vi "t.vi"() -> ()   [LabVIEW 2020]
uses:
  <vilib>/Platform/TimedLoop/XDataNode/timing_clust.ctl
  <vilib>/Platform/TimedLoop/XDataNode/nitl_modes.ctl
  <vilib>/Platform/TimedLoop/XDataNode/wakeup.ctl
  <vilib>/imath/engines/lvmath2/RunTimeEngine/ArithmeticOperatorToken/NIMS_ArithmeticOperator_plus.vi
  <instcachedir>/0/NIMS_ArithmeticOperator_plus_54468E2FAC2848C4BF0D457641184E60.lvgen/NIMS_ArithmeticOperator_plus_54468E2FAC2848C4BF0D457641184E60_012.vi
  <vilib>/imathl/engines/lvmath/Functions/Error Handling/Create Error.vi
  <instcachedir>/0/NIMS_NodeEndStatement_Output_53EC0D466D134D7ABD903AC30B43404B.lvgen/NIMS_NodeEndStatement_Output_53EC0D466D134D7ABD903AC30B43404B_005.vi
  <vilib>/imath/engines/lvmath2/RunTimeEngine/ErrorHandling/NIMS_Finalize Error.vi
  <vilib>/imath/engines/lvmath2/RunTimeEngine/Managers/WorkSpace/UID Generator.vi
  <vilib>/imath/engines/lvmath2/RunTimeEngine/RunTimeType/NIMS_RunTimeType_From StrictType (excl LVString).vi
  <instcachedir>/0/NIMS_RunTimeType_From StrictType (excl LVString)_283B1B2000484AAA8744D21CE97EA49F.lvgen/NIMS_RunTimeType_From StrictType (excl LVString)_283B1B2000484AAA8744D21CE97EA49F_000.vi
  <vilib>/imath/engines/lvmath2/RunTimeEngine/LocalVariableDefStatement/MC_LocalVariableDefStatement_Display.vi
  <vilib>/imath/engines/lvmath2/RunTimeEngine/Managers/SymbolTable/Clear UID.vi
  <instcachedir>/0/NIMS_NodeEndStatement_Output_53EC0D466D134D7ABD903AC30B43404B.lvgen/NIMS_NodeEndStatement_Output_53EC0D466D134D7ABD903AC30B43404B_001.vi
  <instcachedir>/0/NIMS_NodeEndStatement_Output_53EC0D466D134D7ABD903AC30B43404B.lvgen/NIMS_NodeEndStatement_Output_53EC0D466D134D7ABD903AC30B43404B_002.vi
  <vilib>/Platform/TimedLoop/XDataNode/XDataNode.xnode
  <vilib>/Platform/TimedLoop/XDataNode/XDNodeRunTimeDep.lvlib
  <vilib>/imath/engines/lvmath2/RunTimeEngine/Managers/SymbolTable/NIMS_WorkSpace.lvlib
panel:
  in  "保存路径":path=path "C:/Qmz/data1.bin"
  out "Swing":dbl[](graph)
  out "d_next":dbl
  out "y":dbl[][](array[numeric])
  out "添加的数组":dbl[][](array[numeric])
  out "x_next":dbl[](array[numeric])
  out "列数":i32
  out "行数":i32
  out "数组":dbl[](array[numeric])
  in  "PID/ARC":bool
  out "字符串":string="这是开环"
  in  "开环":bool=TRUE
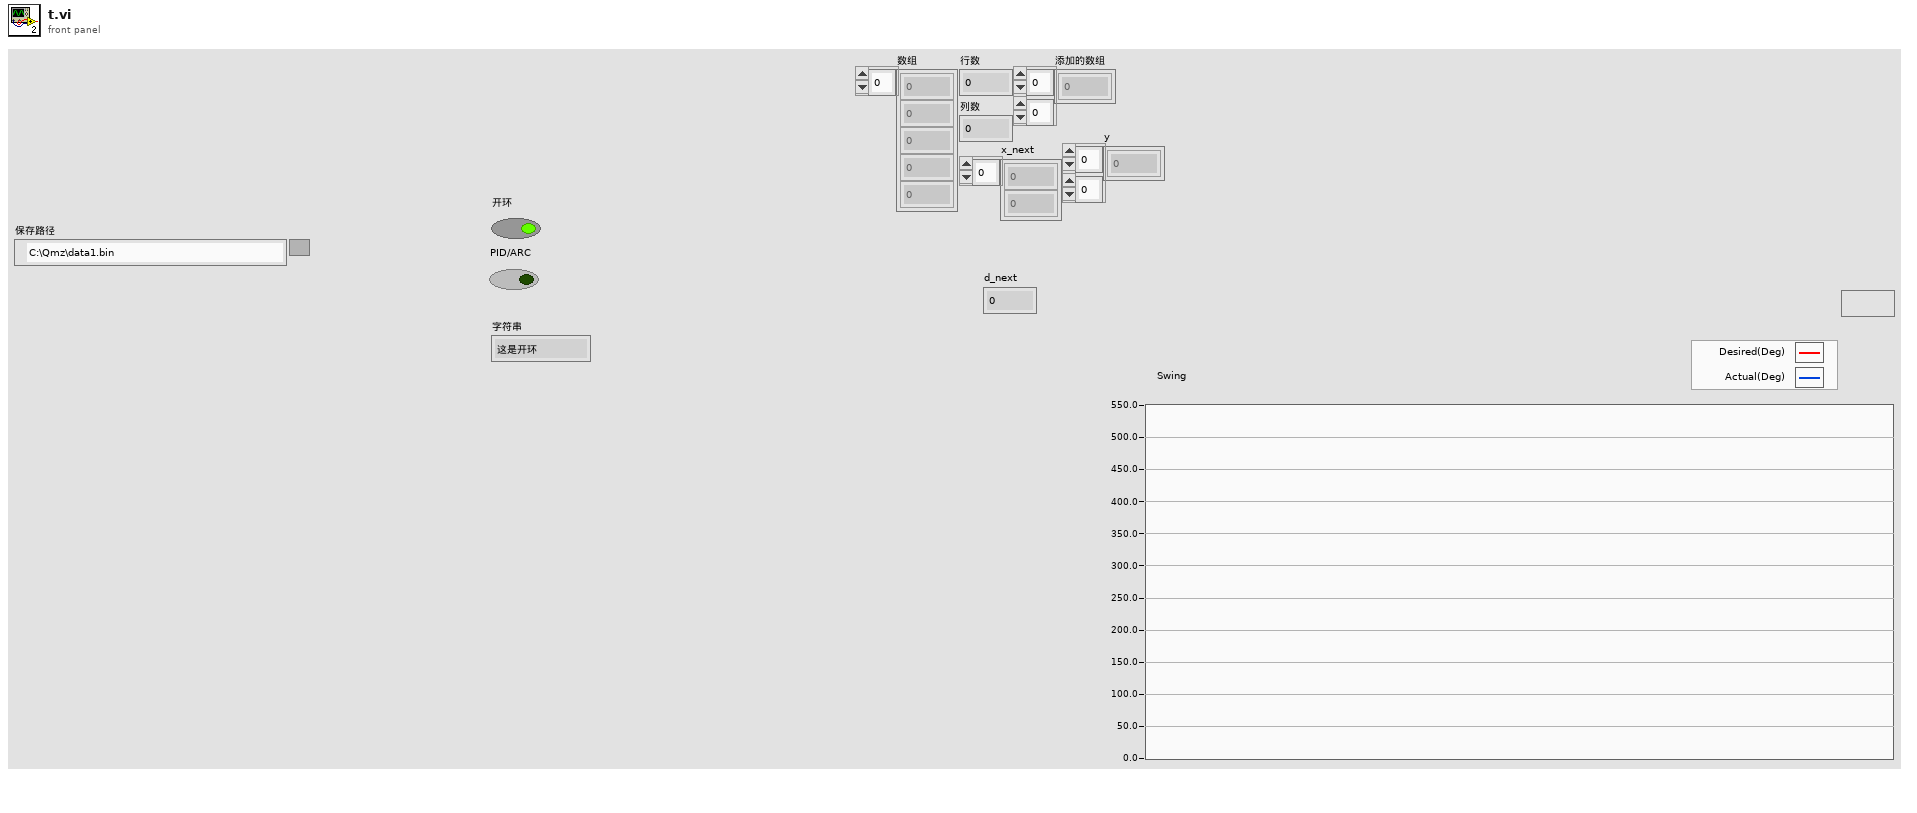
[diagram p1: front panel]
types:
  T1 = enum16{"open", "replace", "create", "open or create", "replace or create", "replace or create with confirmation"}
  T2 = typedef "XDNodeRunTimeDep.lvlib/timing_clust.ctl" = cluster{"Expected End [f-1]":u64, "Actual End [f-1]":u64, "Finished Late? [f-1]":bool, "Expected End [i-1]":u64, "Actual End [i-1]":u64, "Finished Late? [i-1]":bool, "Expected Start [i]":u64, "Actual Start [i]":u64, "Expected Start [f]":u64, "Actual Start [f]":u64, "Source Name":string, "Structure Name":string, "Period":i64, "Deadline":i64, "Offset":i64, "Start":i64, "Priority":i32, "Timeout":i32, "Mode":T3, "Wakeup Reason":T4, "Error":errorcluster, "Source Type":string, "Secondary Source Type":string, "Global End Time":u64, "Global Start Time":u64, "Frame Duration":u64, "Iteration Duration":u64, "Assigned CPU":i32, "I/O Scan Engine Mode":u32}
  T3 = typedef "XDNodeRunTimeDep.lvlib/nitl_modes.ctl" = enum32{"No Change", "Process missed periods, maintain original phase", "Discard missed periods, maintain original phase", "Process missed periods, ignore original phase", "Discard missed periods, ignore original phase"}
  T4 = typedef "XDNodeRunTimeDep.lvlib/wakeup.ctl" = enum32{"Normal", "Aborted", "Asynchronous wakeup", "Timing source error", "Timed loop error", "Timeout"}
  T5 = typedef "NI_Matrix.lvlib/RealMatrix.ctl" = dbl[][]
  T6 = enum16{"big-endian, network order", "native, host order", "little-endian"}
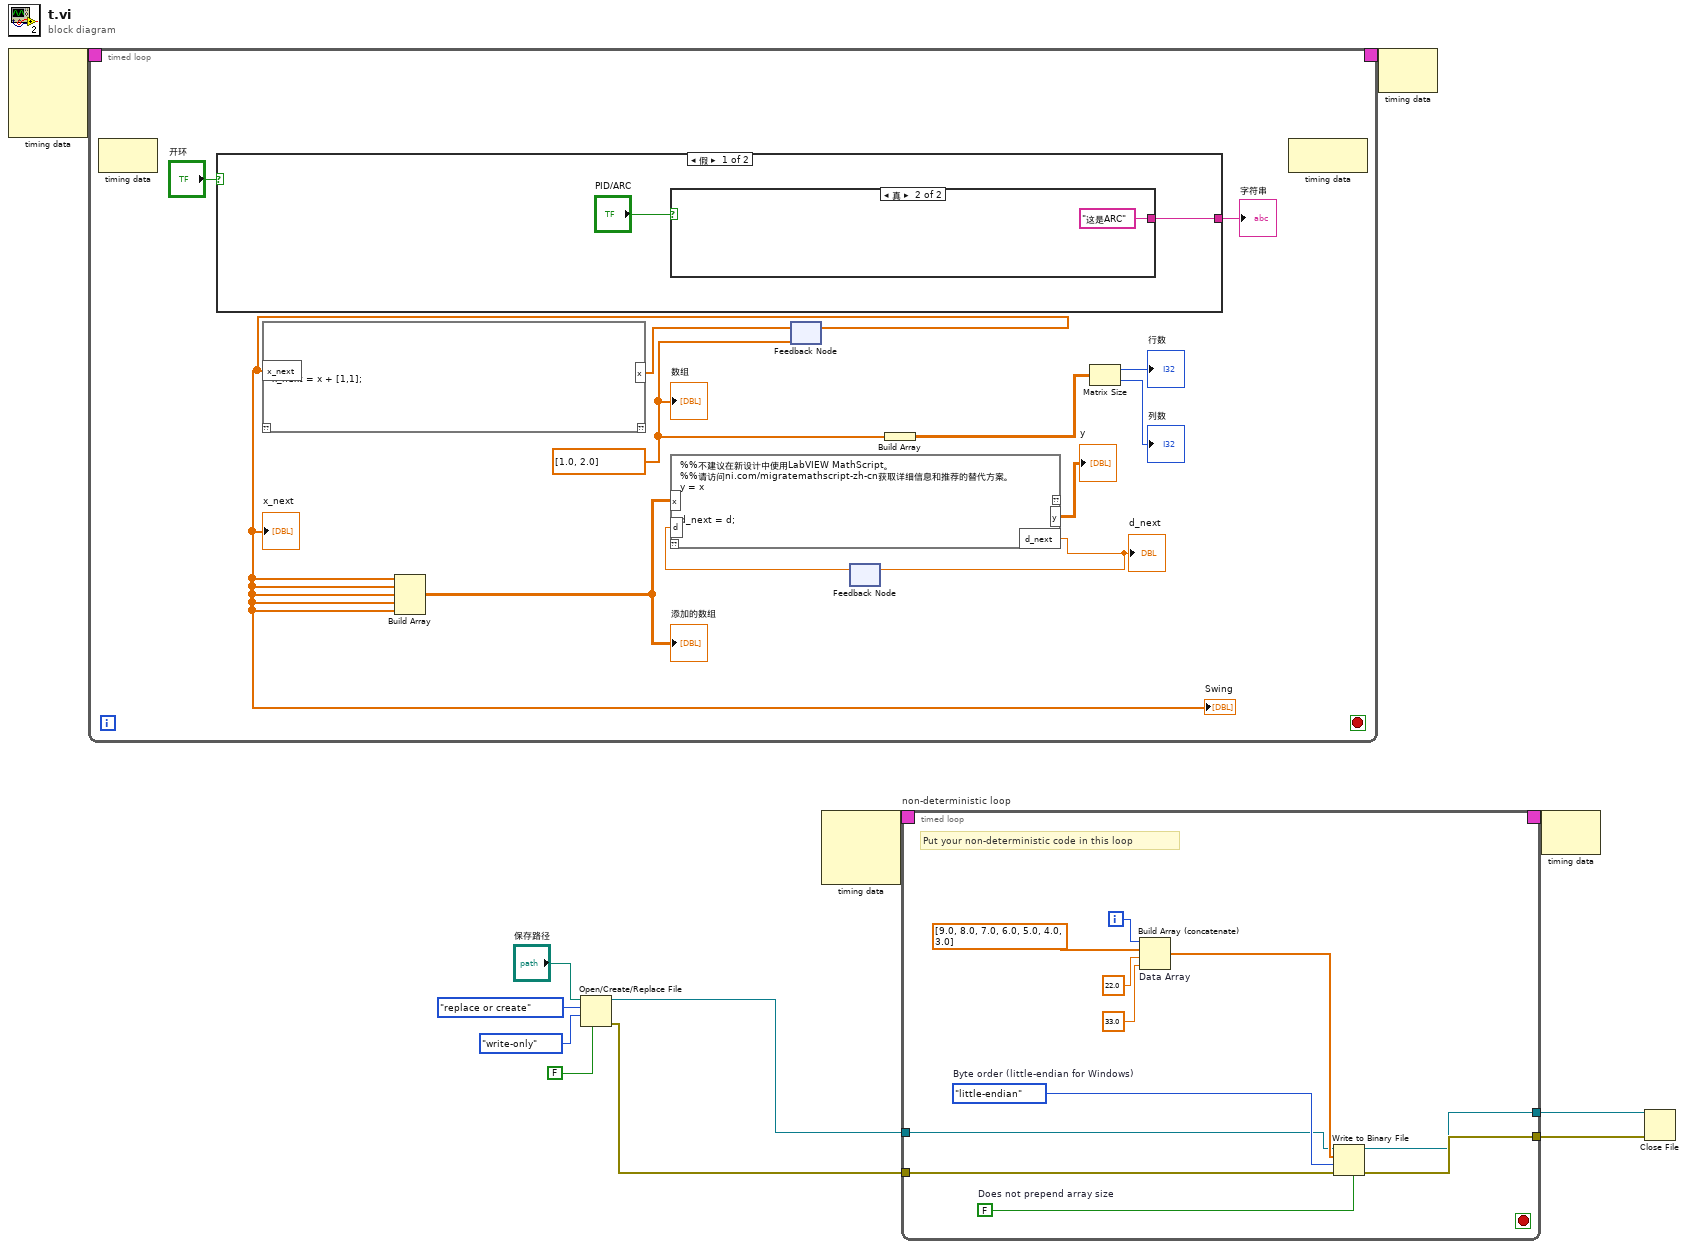
[diagram p0: block diagram]
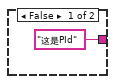
[diagram p2: hidden frame]
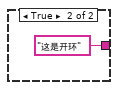
[diagram p3: hidden frame]
diagram:
  n1 = node-c288() -> (w12:T2)  [unwired: 4 in]
  n2 = timed-loop {
    timing: w12 -> [_]
    timing-out: [_] -> w11
    stop <- _ stop-if-true
    w19 = dbl[] [1.0, 2.0]
    n3 = node-c288() -> ()  [unwired: 1 in, 1 out]
    n4 = case shown="假" "开环" {
      tunnel: [w95 "这是开环"] -> w23
      frame False {
        n5 = case shown="真" "PID/ARC" {
          tunnel: ["这是PId" "这是ARC"] -> w95
          frame False {
          }
          frame True {
          }
        }
      }
      frame True {
      }
    }
    "字符串" <- w23
    n6 = feedback #1(w19) -> (w18:dbl[])
    n7 = mathscript code="x_next = x + [1,1];"("x"=w18) -> ("x_next"=w13:dbl[])  [unwired: 1 in, 1 out]
    "x_next" <- w13
    "Swing" <- w13
    n8 = Build Array(w13, w13, w13, w13, w13) -> (w17:dbl[][])
    "添加的数组" <- w17
    n9 = feedback-in #1(w13) -> ()
    n10 = feedback #2() -> (w15:dbl)  [unwired: 1 in]
    n11 = mathscript code="%%不建议在新设计中使用LabVIEW MathScript。\n%%请访问ni.com/migratemathscript-zh-cn获取详细信息和推荐的替代方案。\ny = x\n\n\nd_next = d;"("x"=w17, "d"=w15) -> ("y"=→"y":dbl[][], "d_next"=w14:dbl)  [unwired: 1 in, 1 out]
    "d_next" <- w14
    n12 = feedback-in #2(w14) -> ()
    n13 = Build Array(w19) -> (w22:T5)
    n14 = Matrix Size(0:w22) -> (1:→"行数":i32, 2:→"列数":i32)
    n15 = node-c288() -> ()  [unwired: 1 in, 1 out]
    "数组" <- w19
  }
  n16 = Open/Create/Replace File(file path (use dialog)="保存路径", operation (0:open)=T1."replace or create", access (0:read/write)=enum16{"read/write", "read-only", "write-only"}."write-only" ("权限(0:read/write)"), disable buffering (F)=FALSE) -> (refnum out=w2:refnum<file>, error out=w1:errorcluster)  [unwired: 2 in, 1 out]
  n17 = node-c288 ("Input Node")() -> (w6:T2)  [unwired: 3 in]
  n18 = timed-loop "non-deterministic loop" {
    timing: w6 -> [_]
    timing-out: [_] -> w5
    tunnel: [w111] -> w3
    tunnel: [w110] -> w4
    tunnel: w2 -> [w105]
    tunnel: w1 -> [w104]
    i -> [w109]
    stop <- _ stop-if-true
    w107 = FALSE  # Does not prepend array size
    w108 = T6."little-endian"  # Byte order (little-endian for Windows)
    # "Put your non-deterministic code in this loop"
    n19 = Build Array (concatenate) "Data Array"(w109, dbl[] [9.0, 8.0, 7.0, 6.0, 5.0, 4.0, 3.0], 22.0, 33.0) -> (w106:dbl[])
    n20 = Write to Binary File(file (use dialog)=w105, data=w106, error in=w104, 5:w107, 9:w108) -> (refnum out=w110:refnum<file>, error out=w111:errorcluster)  [unwired: 1 in, 1 out]
  }
  n21 = node-c288(w11) -> ()  [unwired: 1 out]
  n22 = node-c288 ("Output Node")(w5) -> ()  [unwired: 1 out]
  n23 = Close File(refnum=w4, error in=w3) -> ()  [unwired: 2 out]
